vi "DAQ control panel.vi"() -> ()   [LabVIEW 2017]
uses:
  <vilib>/DAQmx/write.llb/DAQmx Write (Analog DBL 1Chan 1Samp).vi
  <vilib>/DAQmx/write.llb/DAQmx Write (Digital Bool 1Line 1Point).vi
  <vilib>/DAQmx/write.llb/DAQmx Write (Analog Wfm 1Chan NSamp).vi
  <vilib>/DAQmx/read.llb/DAQmx Read (Analog 1D DBL 1Chan NSamp).vi
  <vilib>/Analysis/baseanly.llb/Mean (DBL).vi
  <vilib>/DAQmx/read.llb/DAQmx Read (Analog 1D Wfm NChan NSamp).vi
  <vilib>/DAQmx/read.llb/DAQmx Read (Digital Bool 1Line 1Point).vi
  <vilib>/DAQmx/create/channels.llb/DAQmx Create Channel (AO-Voltage-Basic).vi
  <vilib>/DAQmx/miscellaneous.llb/DAQmx Fill In Error Info.vi
  <vilib>/DAQmx/create/channels.llb/DAQmx Create Channel (DO-Digital Output).vi
  <vilib>/DAQmx/create/channels.llb/DAQmx Create Channel (AI-Voltage-Basic).vi
  <vilib>/DAQmx/configure/timing.llb/DAQmx Timing (Sample Clock).vi
  <vilib>/measure/mascope.llb/Amplitude and Levels 1 chan.vi
  <vilib>/measure/mascope.llb/Pulse Measurements 1 chan.vi
  <vilib>/DAQmx/create/channels.llb/DAQmx Create Channel (DI-Digital Input).vi
  <vilib>/measure/NI_MABase.lvlib
  <vilib>/measure/NI_MAPro.lvlib
  <vilib>/Analysis/NI_AALBase.lvlib
panel:
  in  "Expected Input":bool
  out "ao1coerced?":bool caption="Output \nCoerced?"
  out "ao0coerced?":bool caption="Output \nCoerced?"
  in  "Set AO0":bool
  in  "AO0 phase":dbl
  in  "AO0 offset":dbl format="%0.2p"
  in  "AO0 sampling info":cluster{"Samples/sec":dbl, "# of Samples":dbl}={"Samples/sec"=1000000.0, "# of Samples"=1000000.0}
  in  "DC (Ch 0)":bool
  in  "AO0 signal type":T1(ring)
  in  "AO0 Frequency":dbl[unit]=1000.0
  in  "AO0 Amplitude":dbl[unit] min=-10.0 max=10.0
  out "DC offset":dbl[unit]
  out "frequency":dbl[unit]
  out "DC Voltage / Vpp":dbl[unit] format="%.2p"
  out "period":dbl[unit] format="%.2g"
  in  "# of samples":i32=1000
  in  "rate":dbl[unit]=1000.0 format="%0.2f"
  out "data":waveform(dbl)(graph)
  out "Digital Inputs":bool[](array[boolean])
  in  "Read Digital":bool
  in  "Digital toggle":bool[](array[boolean])=[FALSE, FALSE, FALSE, FALSE, FALSE, FALSE, FALSE, FALSE]
  in  "Digital Outputs":bool[](array[boolean])=[FALSE, FALSE, FALSE, FALSE, FALSE, FALSE, FALSE, FALSE]
  in  "physical channels":tag="Dev1/ai0"
  in  "Read Analog":bool
  in  "Set AO1":bool
  in  "AO1 phase":dbl
  in  "AO1 offset":dbl format="%0.2p"
  in  "AO1 sampling info":cluster{"Samples/sec":dbl, "# of Samples":dbl}={"Samples/sec"=1000000.0, "# of Samples"=1000000.0}
  in  "DC (Ch 1)":bool
  out "error out":errorcluster
  in  "error in (no error)":errorcluster
  in  "AO1 signal type":T1(ring)
  in  "AO1 Frequency":dbl[unit]=1000.0
  in  "AO1 Amplitude":dbl[unit] min=-10.0 max=10.0
  in  "stop":bool
  # "BNC-2120"
  # "7"
  # "7"
  # "7"
  # "6"
  # "6"
  # "6"
  # "5"
  # "5"
  # "5"
  # "AC"
  # "4"
  # "4"
  # "4"
  # "3"
  # "3"
  # "3"
  # "2"
  # "2"
  # "2"
  # "1"
  # "1"
  # "1"
  # "0"
  # "0"
  # "0"
  # "Output"
  # "Input"
  # "AC"
  # "DC"
  # "AC"
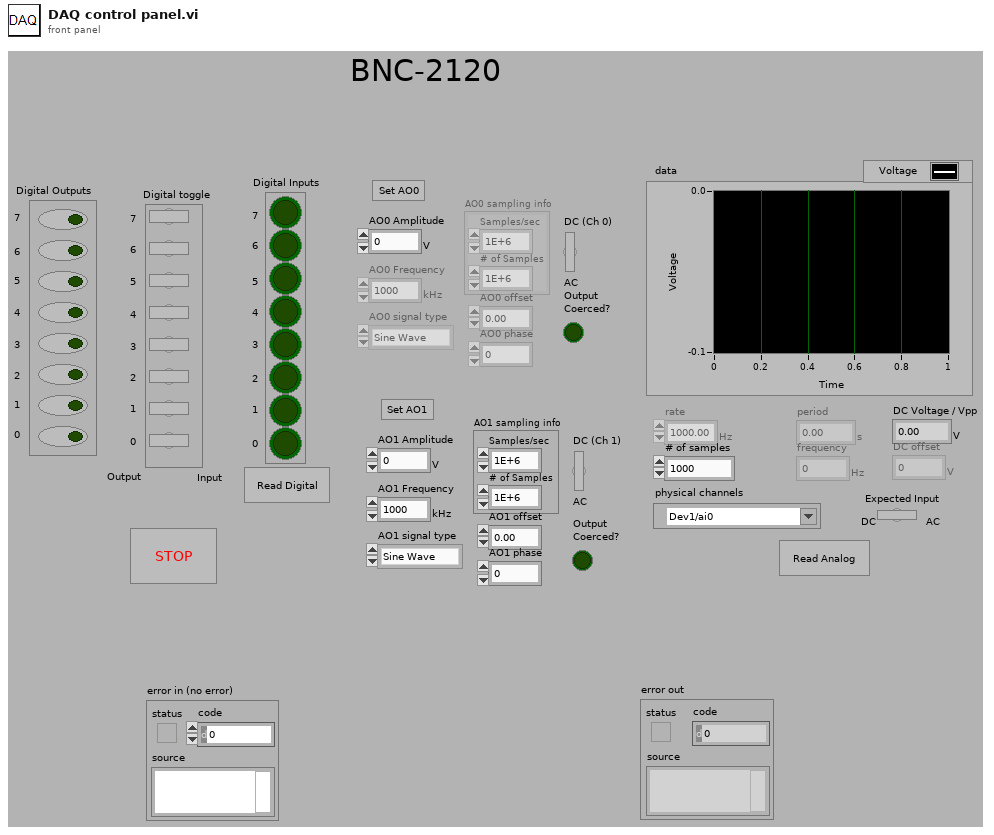
[diagram p1: front panel]
types:
  T1 = enum16{"Sine Wave", "Triangle Wave", "Square Wave", "Sawtooth Wave"}
  T2 = cluster{"AO ch0":refnum<k21>, "AO ch1":refnum<k21>}
  T3 = enum8{"Enabled", "Disabled", "Disabled and Grayed Out"}
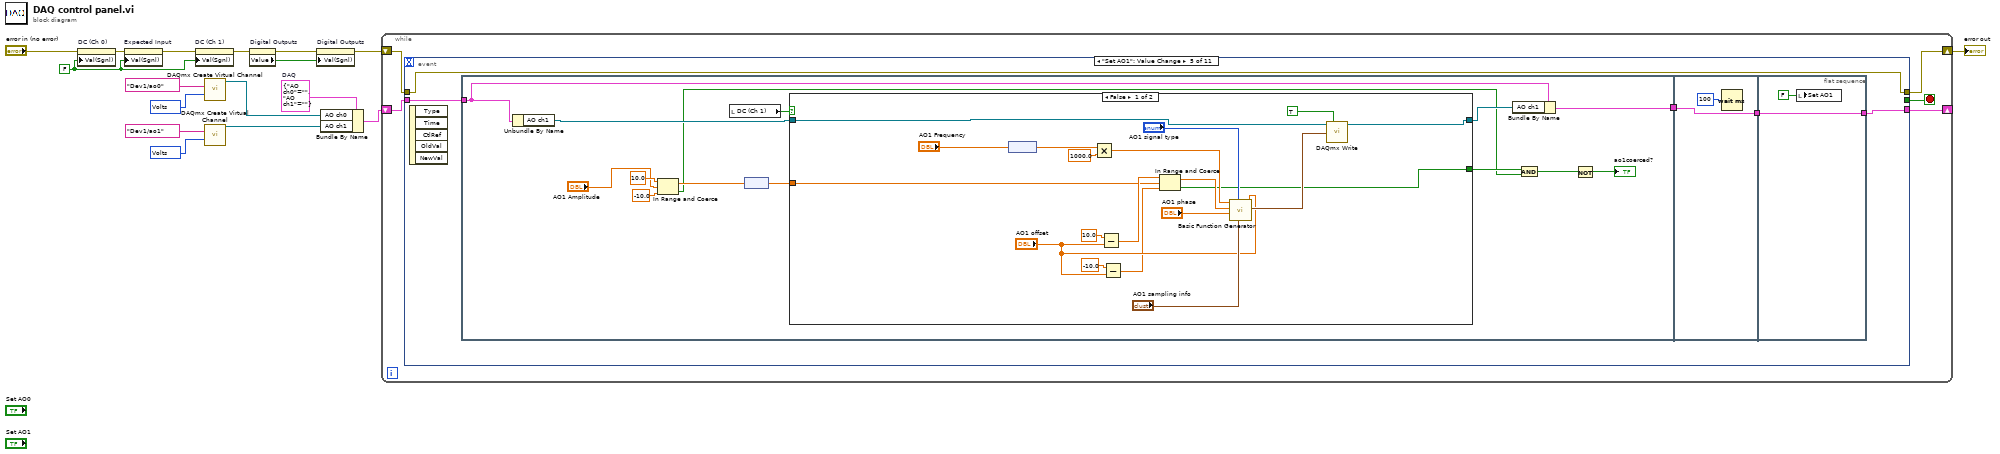
[diagram p0: block diagram]
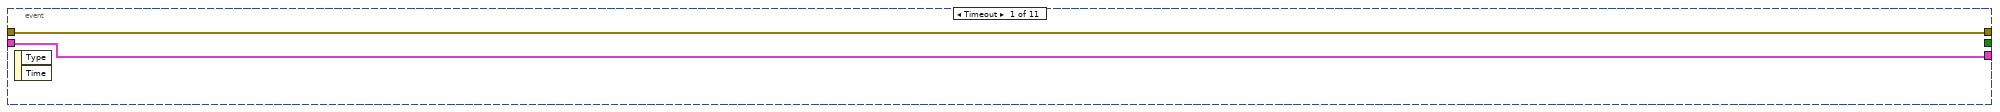
[diagram p2: hidden frame]
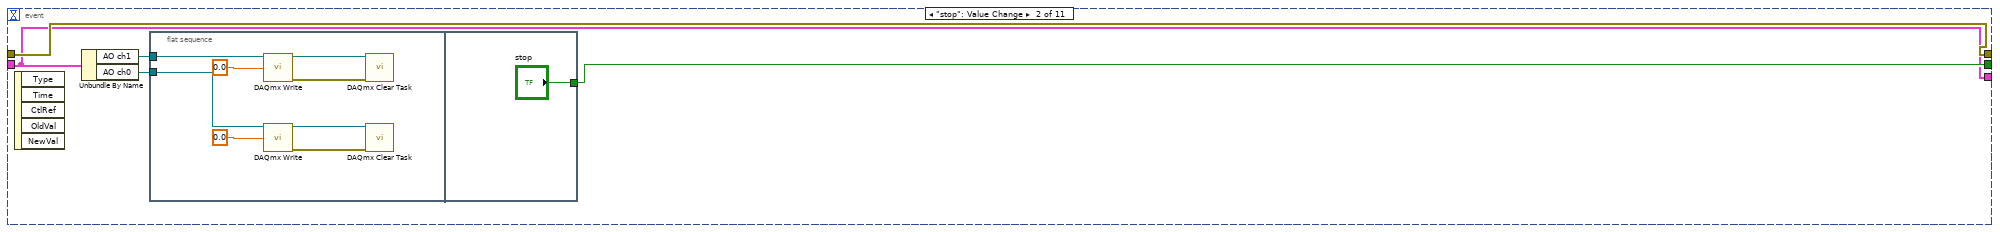
[diagram p3: hidden frame]
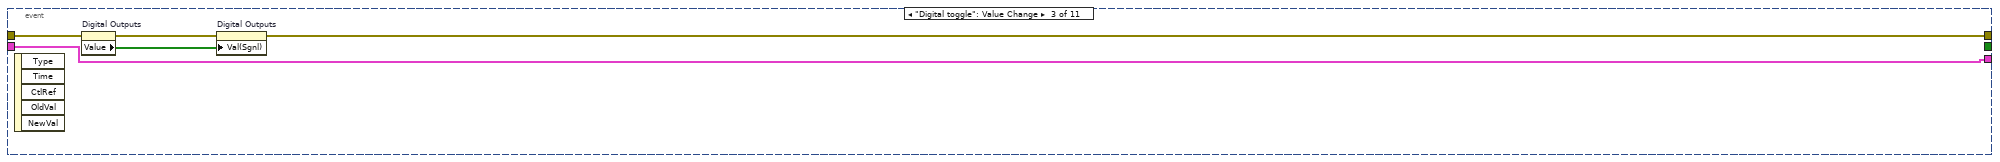
[diagram p4: hidden frame]
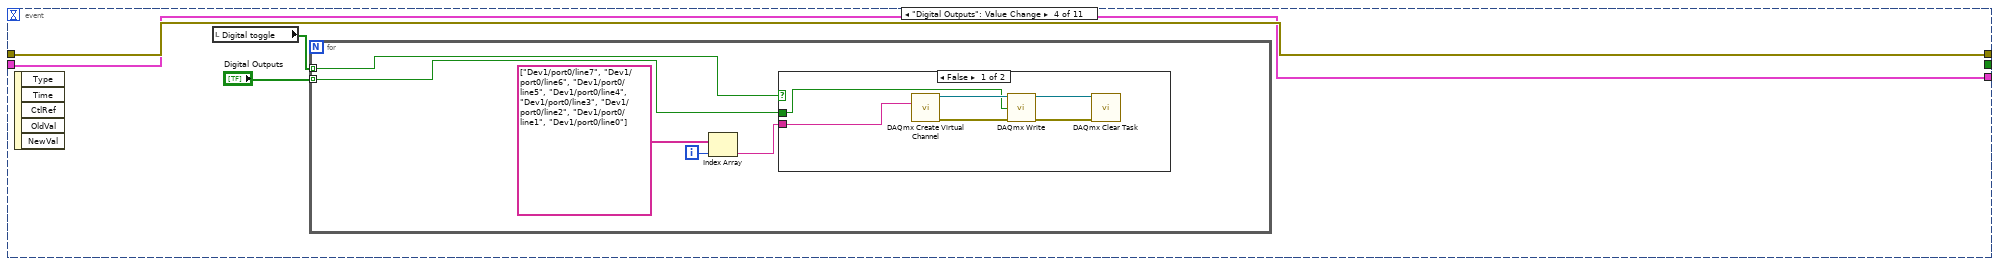
[diagram p5: hidden frame]
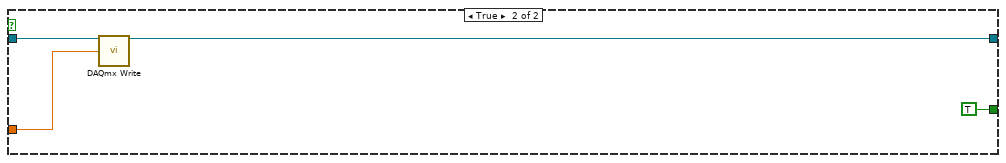
[diagram p7: hidden frame]
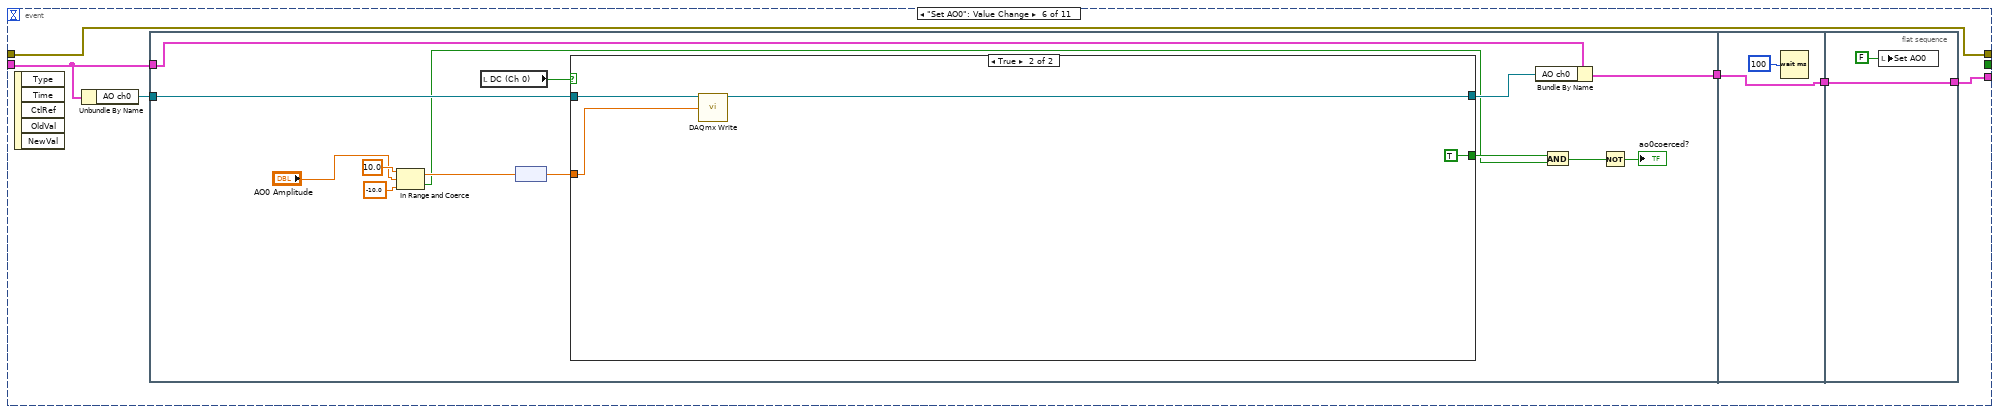
[diagram p8: hidden frame]
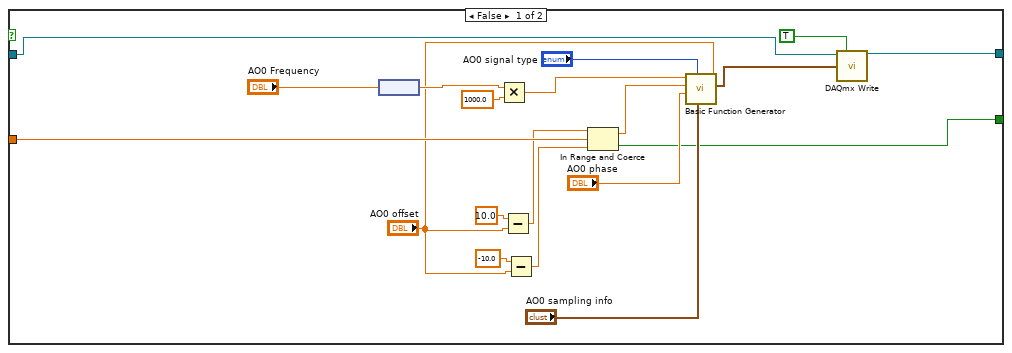
[diagram p9: hidden frame]
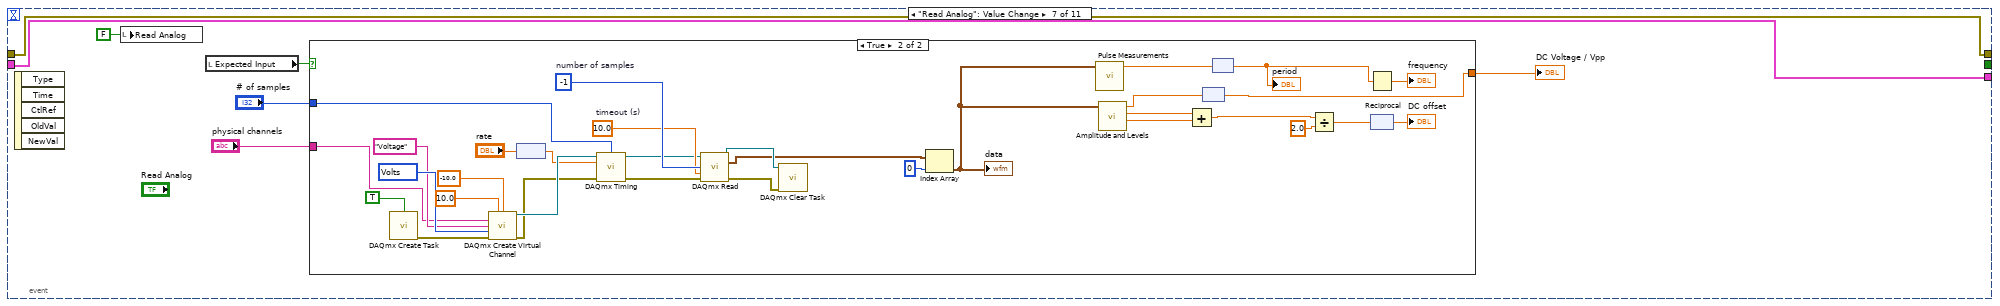
[diagram p10: hidden frame]
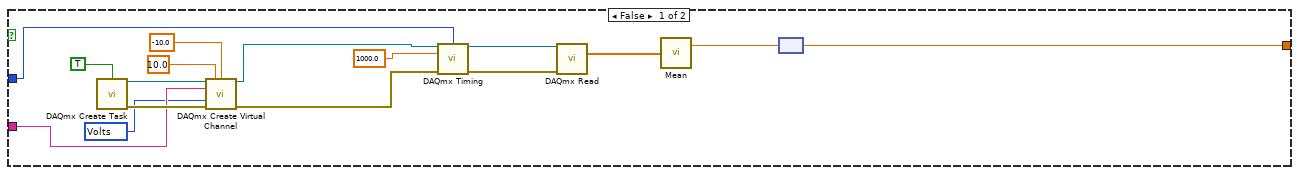
[diagram p11: hidden frame]
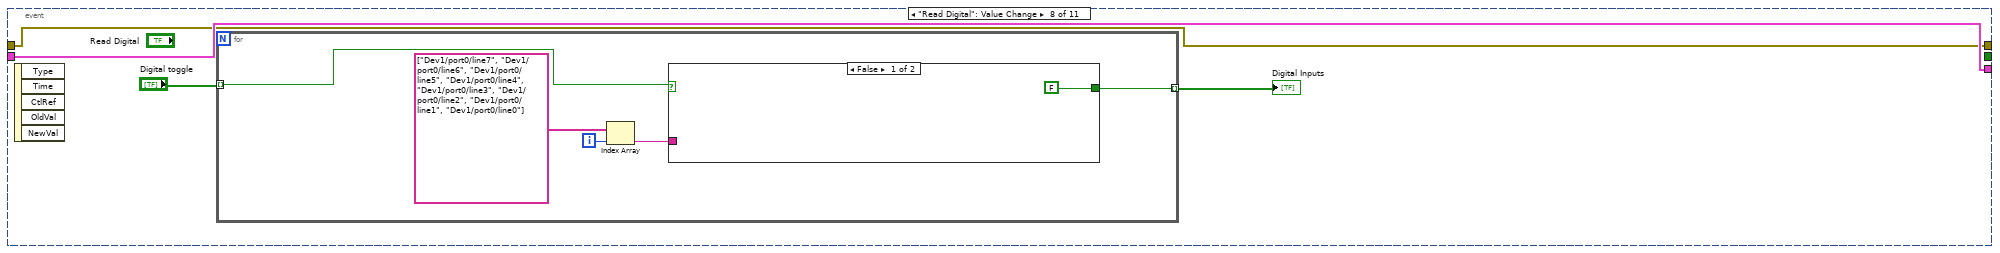
[diagram p12: hidden frame]
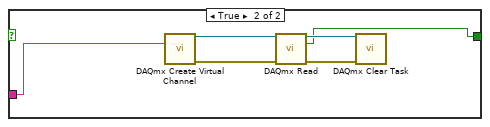
[diagram p13: hidden frame]
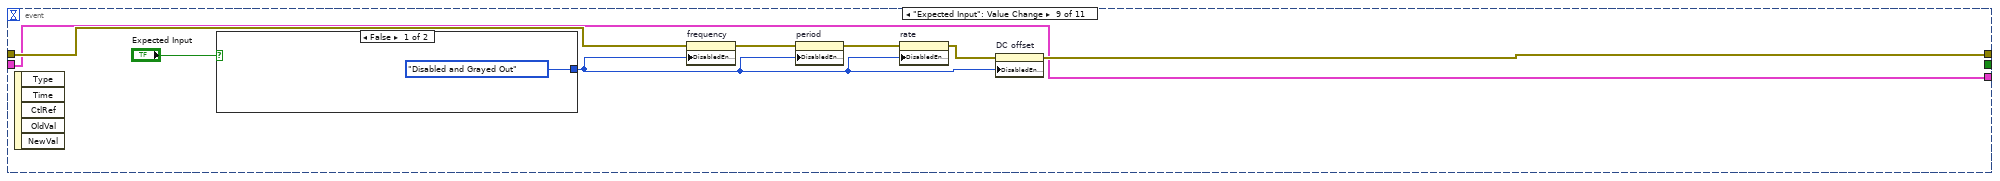
[diagram p14: hidden frame]
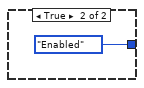
[diagram p15: hidden frame]
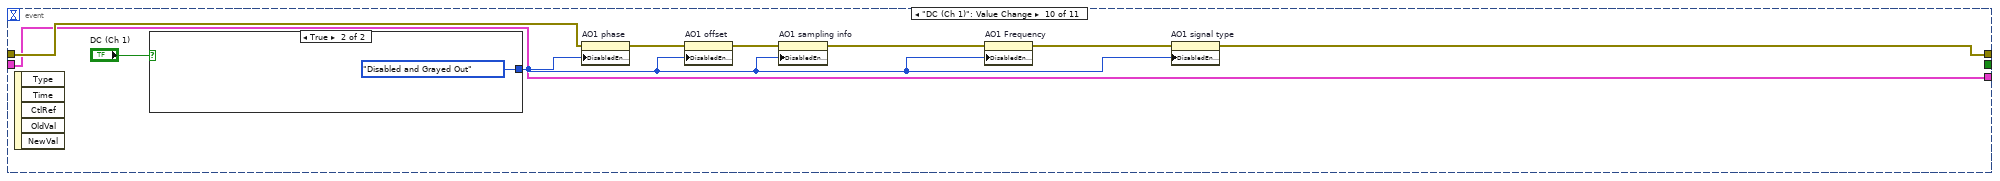
[diagram p16: hidden frame]
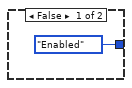
[diagram p17: hidden frame]
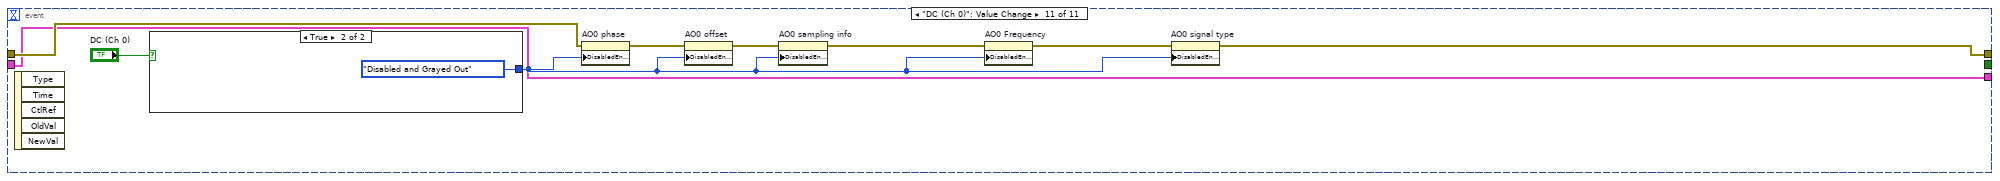
[diagram p18: hidden frame]
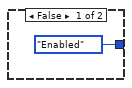
[diagram p19: hidden frame]
diagram:
  w12 = T2 {"AO ch0"="", "AO ch1"=""}  # DAQ
  w13 = 10348 items=["Volts"=10348, "From Custom Scale"=10065] ("units")
  w16 = 10348 items=["Volts"=10348, "From Custom Scale"=10065] ("units")
  w5 = FALSE ("DC (Ch 0)")
  n1 = property on="DC (Ch 0)" class="Bool (strict)"(error in="error in (no error)", "Val(Sgnl)"=w5) -> (error out=w6:errorcluster)  [unwired: 1 in, 1 out]
  n2 = property on="Expected Input" class="Bool (strict)"(error in=w6, "Val(Sgnl)"=w5) -> (error out=w7:errorcluster)  [unwired: 1 in, 1 out]
  n3 = property on="DC (Ch 1)" class="Bool (strict)"(error in=w7, "Val(Sgnl)"=w5) -> (error out=w2:errorcluster)  [unwired: 1 in, 1 out]
  n4 = call-poly <vilib>:"DAQmx Create Virtual Channel.vi"("physical channels"=tag "Dev1/ao0", "units"=w16) -> ("task out"=w10:refnum<k21>)  [unwired: 12 in, 1 out]
  n5 = call-poly <vilib>:"DAQmx Create Virtual Channel.vi"("physical channels"=tag "Dev1/ao1", "units"=w13) -> ("task out"=w11:refnum<k21>)  [unwired: 12 in, 1 out]
  n6 = property on="Digital Outputs" class="Arr (strict)"(error in=w2) -> (error out=w3:errorcluster, "Value"=w4:bool[])  [unwired: 1 in, 1 out]
  n7 = property on="Digital Outputs" class="Arr (strict)"(error in=w3, "Val(Sgnl)"=w4) -> (error out=w1:errorcluster)  [unwired: 1 in, 1 out]
  n8 = Bundle By Name(cluster=w12, "AO ch0"=w10, "AO ch1"=w11) -> (w9:T2)
  n9 = while {
    shift-right: [w20] -> w17
    shift-left: w1 -> [w21]
    shift-right: [w18] -> _
    shift-left: w9 -> [w19]
    stop <- w22 stop-if-true
    n10 = event shown="[4] \"Set AO1\": Value Change" {
      selector: _ -> [_ _ _ _ _ _ _ _ _ _ _]
      dyn-events: _ -> [_ _ _ _ _ _ _ _ _ _ _]
      timeout: _ -> [_ _ _ _ _ _ _ _ _ _ _]
      tunnel: [_ w29 _ _ _ _ _ _ _ _ _] -> w22
      tunnel: w21 -> [w24 w28 w40 w47 w63 w110 w157 w207 w230 w236 w247]
      tunnel: [w24 w28 w39 w47 w63 w110 w157 w207 w225 w237 w248] -> w20
      tunnel: w19 -> [w23 w27 w43 w44 w62 w108 w158 w208 w223 w234 w245]
      tunnel: [w23 w27 w43 w44 w61 w107 w158 w208 w223 w234 w245] -> w18
      event Timeout {
        n11 = event-data() -> ()  [unwired: 1 in, 2 out]
      }
      event "stop": Value Change {
        n12 = event-data() -> ()  [unwired: 1 in, 5 out]
        n13 = Unbundle By Name(w27) -> ("AO ch1"=w26:refnum<k21>, "AO ch0"=w25:refnum<k21>)
        n14 = flat-sequence {
          tunnel: w26 -> [w34]
          tunnel: w25 -> [w30]
          tunnel: ["stop"] -> w29
          frame #0 {
            n15 = call-poly <vilib>:"DAQmx Write.vi"("task/channels in"=w34, "data"=0.0) -> ("task out"=w37:refnum<k21>, "error out"=w36:errorcluster)  [unwired: 11 in, 1 out]
            n16 = call-poly <vilib>:"DAQmx Write.vi"("task/channels in"=w30, "data"=0.0) -> ("task out"=w31:refnum<k21>, "error out"=w32:errorcluster)  [unwired: 11 in, 1 out]
            n17 = call <vilib>:"DAQmx Clear Task.vi"("task in"=w37, "error in"=w36) -> ()  [unwired: 13 in, 1 out]
            n18 = call <vilib>:"DAQmx Clear Task.vi"("task in"=w31, "error in"=w32) -> ()  [unwired: 13 in, 1 out]
          }
          frame #1 {
          }
        }
      }
      event "Digital toggle": Value Change {
        n19 = event-data() -> ()  [unwired: 1 in, 5 out]
        n20 = property on="Digital Outputs" class="Arr (strict)"(error in=w40) -> (error out=w41:errorcluster, "Value"=w42:bool[])  [unwired: 1 in, 1 out]
        n21 = property on="Digital Outputs" class="Arr (strict)"(error in=w41, "Val(Sgnl)"=w42) -> (error out=w39:errorcluster)  [unwired: 1 in, 1 out]
      }
      event "Digital Outputs": Value Change {
        n22 = event-data() -> ()  [unwired: 1 in, 5 out]
        n23 = local read "Digital toggle"() -> (w45:bool[])
        n24 = for {
          tunnel: "Digital Outputs" -> [w48] mode=indexing
          tunnel: w45 -> [w49] mode=indexing
          i -> [w51]
          n25 = Index Array(array=tag[] ["Dev1/port0/line7", "Dev1/port0/line6", "Dev1/port0/line5", "Dev1/port0/line4", "Dev1/port0/line3", "Dev1/port0/line2", "Dev1/port0/line1", "Dev1/port0/line0"], index=w51) -> (element=w50:tag)
          n26 = case shown="False" w49 {
            tunnel: w50 -> [w58 _]
            tunnel: w48 -> [w55 _]
            frame False {
              n27 = call-poly <vilib>:"DAQmx Create Virtual Channel.vi"("lines"=w58) -> ("task out"=w57:refnum<k21>, "error out"=w56:errorcluster)  [unwired: 13 in]
              n28 = call-poly <vilib>:"DAQmx Write.vi"("task/channels in"=w57, "data"=w55, "error in"=w56) -> ("task out"=w54:refnum<k21>, "error out"=w53:errorcluster)  [unwired: 10 in, 1 out]
              n29 = call <vilib>:"DAQmx Clear Task.vi"("task in"=w54, "error in"=w53) -> ()  [unwired: 13 in, 1 out]
            }
            frame True {
            }
          }
        }
      }
      event "Set AO1": Value Change {
        n30 = event-data() -> ()  [unwired: 1 in, 5 out]
        n31 = flat-sequence {
          tunnel: w62 -> [w72]
          tunnel: [w71] -> w60
          tunnel: w60 -> [w102]
          tunnel: [w102] -> w59
          tunnel: [w104] -> w61
          tunnel: w59 -> [w104]
          frame #0 {
            n32 = Unbundle By Name(w72) -> ("AO ch1"=w76:refnum<k21>)
            n33 = In Range and Coerce(upper limit=dbl[unit] 10.0, x="AO1 Amplitude", lower limit=dbl[unit] -10.0) -> (coerced(x)=w73:dbl[unit], In Range?=w64:bool)
            n34 = local read "DC (Ch 1)"() -> (w68:bool)
            n35 = node(w73) -> (w77:dbl)
            n36 = case shown="False" w68 {
              tunnel: w76 -> [w78 w100]
              tunnel: w77 -> [w83 w99]
              tunnel: [w89 w98] -> w70
              tunnel: [w79 TRUE] -> w65
              frame False {
                n37 = node("AO1 Frequency") -> (w95:dbl)
                n38 = Multiply(x=w95, y=1000.0) -> (x*y=w87:dbl)
                n39 = Subtract(x=10.0, y="AO1 offset") -> (x-y=w86:dbl)
                n40 = Subtract(x=-10.0, y="AO1 offset") -> (x-y=w81:dbl)
                n41 = In Range and Coerce(upper limit=w86, x=w83, lower limit=w81) -> (coerced(x)=w80:dbl, In Range?=w79:bool)
                n42 = call <vilib>:"Basic Function Generator.vi"("offset"="AO1 offset", "sampling info"="AO1 sampling info", "signal type"="AO1 signal type", "phase"="AO1 phase", "amplitude"=w80, "frequency"=w87) -> ("signal out"=w94:waveform(dbl))  [unwired: 3 in, 2 out]
                n43 = call-poly <vilib>:"DAQmx Write.vi"("task/channels in"=w78, "auto start"=TRUE, "data"=w94) -> ("task out"=w89:refnum<k21>)  [unwired: 10 in, 2 out]
              }
              frame True {
                n44 = call-poly <vilib>:"DAQmx Write.vi"("task/channels in"=w100, "data"=w99) -> ("task out"=w98:refnum<k21>)  [unwired: 11 in, 2 out]
              }
            }
            n45 = Bundle By Name(cluster=w72, "AO ch1"=w70) -> (w71:T2)
            n46 = And(x=w65, y=w64) -> (x .and. y?=w66:bool)
            n47 = Not(x=w66) -> (.not. x?=→"ao1coerced?":bool)
          }
          frame #1 {
            n48 = Wait (ms)(milliseconds to wait=u32 100) -> ()  [unwired: 1 out]
          }
          frame #2 {
            n49 = local write "Set AO1"(FALSE ("Set AO1")) -> ()
          }
        }
      }
      event "Set AO0": Value Change {
        n50 = event-data() -> ()  [unwired: 1 in, 5 out]
        n51 = Unbundle By Name(w108) -> ("AO ch0"=w109:refnum<k21>)
        n52 = flat-sequence {
          tunnel: w109 -> [w123]
          tunnel: w108 -> [w119]
          tunnel: [w118] -> w106
          tunnel: w106 -> [w149]
          tunnel: [w149] -> w105
          tunnel: [w151] -> w107
          tunnel: w105 -> [w151]
          frame #0 {
            n53 = In Range and Coerce(upper limit=dbl[unit] 10.0, x="AO0 Amplitude", lower limit=dbl[unit] -10.0) -> (coerced(x)=w120:dbl[unit], In Range?=w113:bool)
            n54 = local read "DC (Ch 0)"() -> (w115:bool)
            n55 = node(w120) -> (w124:dbl)
            n56 = case shown="True" w115 {
              tunnel: w123 -> [w139 w147]
              tunnel: w124 -> [w132 w146]
              tunnel: [w138 w145] -> w117
              tunnel: [w125 TRUE] -> w114
              frame False {
                n57 = node("AO0 Frequency") -> (w142:dbl)
                n58 = Multiply(x=w142, y=1000.0) -> (x*y=w133:dbl)
                n59 = Subtract(x=10.0, y="AO0 offset") -> (x-y=w131:dbl)
                n60 = Subtract(x=-10.0, y="AO0 offset") -> (x-y=w129:dbl)
                n61 = In Range and Coerce(upper limit=w131, x=w132, lower limit=w129) -> (coerced(x)=w126:dbl, In Range?=w125:bool)
                n62 = call <vilib>:"Basic Function Generator.vi"("offset"="AO0 offset", "sampling info"="AO0 sampling info", "signal type"="AO0 signal type", "phase"="AO0 phase", "amplitude"=w126, "frequency"=w133) -> ("signal out"=w141:waveform(dbl))  [unwired: 3 in, 2 out]
                n63 = call-poly <vilib>:"DAQmx Write.vi"("task/channels in"=w139, "auto start"=TRUE, "data"=w141) -> ("task out"=w138:refnum<k21>)  [unwired: 10 in, 2 out]
              }
              frame True {
                n64 = call-poly <vilib>:"DAQmx Write.vi"("task/channels in"=w147, "data"=w146) -> ("task out"=w145:refnum<k21>)  [unwired: 11 in, 2 out]
              }
            }
            n65 = Bundle By Name(cluster=w119, "AO ch0"=w117) -> (w118:T2)
            n66 = And(x=w114, y=w113) -> (x .and. y?=w112:bool)
            n67 = Not(x=w112) -> (.not. x?=→"ao0coerced?":bool)
          }
          frame #1 {
            n68 = Wait (ms)(milliseconds to wait=u32 100) -> ()  [unwired: 1 out]
          }
          frame #2 {
            n69 = local write "Set AO0"(FALSE ("Set AO1")) -> ()
          }
        }
      }
      event "Read Analog": Value Change {
        n70 = event-data() -> ()  [unwired: 1 in, 5 out]
        n71 = local write "Read Analog"(FALSE ("Read AI")) -> ()
        n72 = local read "Expected Input"() -> (w153:bool)
        n73 = case shown="True" w153 {
          tunnel: "physical channels" -> [w167 w177]
          tunnel: [w160 w176] -> w154
          tunnel: "# of samples" -> [w159 w175]
          frame False {
            w162 = 10348 items=["Volts"=10348, "From Custom Scale"=10065] ("units")
            n74 = call <vilib>:"DAQmx Create Task.vi"("auto cleanup"=TRUE) -> ("task out"=w173:refnum<k21>, "error out"=w170:errorcluster)  [unwired: 13 in]
            n75 = call-poly <vilib>:"DAQmx Create Virtual Channel.vi"("task in"=w173, "maximum value"=10.0, "minimum value"=-10.0, "physical channels"=w167, "units"=w162, "error in"=w170) -> ("task out"=w169:refnum<k21>, "error out"=w168:errorcluster)  [unwired: 8 in]
            n76 = call-poly <vilib>:"DAQmx Timing.vi"("task/channels in"=w169, "samples per channel"=w159, "rate"=1000.0, "error in"=w168) -> ("task out"=w165:refnum<k21>, "error out"=w164:errorcluster)  [unwired: 10 in]
            n77 = call-poly <vilib>:"DAQmx Read.vi"("task/channels in"=w165, "error in"=w164) -> ("data"=w163:dbl[])  [unwired: 11 in, 2 out]
            n78 = call-poly <vilib>:"Mean.vi"("X"=w163) -> ("mean"=w161:dbl)  [unwired: 1 out]
            n79 = node(w161) -> (w160:dbl[unit])
          }
          frame True {
            w200 = 10348 items=["Volts"=10348, "From Custom Scale"=10065] ("units")
            w205 = 10.0  # timeout (s)
            w206 = -1  # number of samples
            n80 = call <vilib>:"DAQmx Create Task.vi"("auto cleanup"=TRUE) -> ("error out"=w201:errorcluster)  [unwired: 13 in, 1 out]
            n81 = call-poly <vilib>:"DAQmx Create Virtual Channel.vi"("maximum value"=10.0, "minimum value"=-10.0, "physical channels"=w177, "name to assign"="Voltage", "units"=w200, "error in"=w201) -> ("task out"=w196:refnum<k21>, "error out"=w195:errorcluster)  [unwired: 8 in]
            n82 = node("rate") -> (w186:dbl)
            n83 = call-poly <vilib>:"DAQmx Timing.vi"("task/channels in"=w196, "samples per channel"=w175, "rate"=w186, "error in"=w195) -> ("task out"=w194:refnum<k21>, "error out"=w193:errorcluster)  [unwired: 10 in]
            n84 = call-poly <vilib>:"DAQmx Read.vi"("task/channels in"=w194, "number of samples per channel"=w206, "timeout"=w205, "error in"=w193) -> ("task out"=w203:refnum<k21>, "data"=w192:waveform(dbl)[], "error out"=w204:errorcluster)  [unwired: 9 in]
            n85 = call <vilib>:"DAQmx Clear Task.vi"("task in"=w203, "error in"=w204) -> ()  [unwired: 13 in, 1 out]
            n86 = Index Array(array=w192, index=0) -> (element=w190:waveform(dbl))
            "data" <- w190
            n87 = call-poly <vilib>:"Pulse Measurements.vi"("signal in"=w190) -> ("period"=w189:dbl)  [unwired: 6 in, 4 out]
            n88 = call-poly <vilib>:"Amplitude and Levels.vi"("signal in"=w190) -> ("low state level"=w182:dbl, "high state level"=w183:dbl, "amplitude"=w188:dbl)  [unwired: 7 in, 1 out]
            n89 = Add(x=w183, y=w182) -> (x+y=w181:dbl)
            n90 = node(w188) -> (w176:dbl[unit])
            n91 = node(w189) -> (w185:dbl[unit])
            "period" <- w185
            n92 = Divide(x=w181, y=2.0) -> (x/y=w179:dbl)
            n93 = Reciprocal(x=w185) -> (1/x=→"frequency":dbl[unit])
            n94 = node(w179) -> (→"DC offset":dbl[unit])
          }
        }
        "DC Voltage / Vpp" <- w154
      }
      event "Read Digital": Value Change {
        n95 = event-data() -> ()  [unwired: 1 in, 5 out]
        n96 = for {
          tunnel: "Digital toggle" -> [w211] mode=indexing
          tunnel: [w212] -> w209 mode=indexing
          i -> [w214]
          n97 = Index Array(array=tag[] ["Dev1/port0/line7", "Dev1/port0/line6", "Dev1/port0/line5", "Dev1/port0/line4", "Dev1/port0/line3", "Dev1/port0/line2", "Dev1/port0/line1", "Dev1/port0/line0"], index=w214) -> (element=w213:tag)
          n98 = case shown="False" w211 {
            tunnel: w213 -> [_ w221]
            tunnel: [FALSE w217] -> w212
            frame False {
            }
            frame True {
              n99 = call-poly <vilib>:"DAQmx Create Virtual Channel.vi"("lines"=w221) -> ("task out"=w222:refnum<k21>, "error out"=w220:errorcluster)  [unwired: 13 in]
              n100 = call-poly <vilib>:"DAQmx Read.vi"("task/channels in"=w222, "error in"=w220) -> ("task out"=w218:refnum<k21>, "data"=w217:bool, "error out"=w219:errorcluster)  [unwired: 11 in]
              n101 = call <vilib>:"DAQmx Clear Task.vi"("task in"=w218, "error in"=w219) -> ()  [unwired: 13 in, 1 out]
            }
          }
        }
        "Digital Inputs" <- w209
      }
      event "Expected Input": Value Change {
        n102 = event-data() -> ()  [unwired: 1 in, 5 out]
        n103 = case shown="False" "Expected Input" {
          tunnel: [T3."Disabled and Grayed Out" ("Disabled") T3."Enabled" ("Disabled")] -> w226
          frame False {
          }
          frame True {
          }
        }
        n104 = property on="frequency" class="DigNum (strict)"(error in=w230, "DisabledEnum"=w226) -> (error out=w229:errorcluster)  [unwired: 1 in, 1 out]
        n105 = property on="period" class="DigNum (strict)"(error in=w229, "DisabledEnum"=w226) -> (error out=w228:errorcluster)  [unwired: 1 in, 1 out]
        n106 = property on="rate" class="DigNum (strict)"(error in=w228, "DisabledEnum"=w226) -> (error out=w227:errorcluster)  [unwired: 1 in, 1 out]
        n107 = property on="DC offset" class="DigNum (strict)"(error in=w227, "DisabledEnum"=w226) -> (error out=w225:errorcluster)  [unwired: 1 in, 1 out]
      }
      event "DC (Ch 1)": Value Change {
        n108 = event-data() -> ()  [unwired: 1 in, 5 out]
        n109 = case shown="True" "DC (Ch 1)" {
          tunnel: [T3."Enabled" ("Disabled") T3."Disabled and Grayed Out" ("Disabled")] -> w235
          frame False {
          }
          frame True {
          }
        }
        n110 = property on="AO1 phase" class="DigNum (strict)"(error in=w236, "DisabledEnum"=w235) -> (error out=w238:errorcluster)  [unwired: 1 in, 1 out]
        n111 = property on="AO1 offset" class="DigNum (strict)"(error in=w238, "DisabledEnum"=w235) -> (error out=w239:errorcluster)  [unwired: 1 in, 1 out]
        n112 = property on="AO1 sampling info" class="Clust (strict)"(error in=w239, "DisabledEnum"=w235) -> (error out=w240:errorcluster)  [unwired: 1 in, 1 out]
        n113 = property on="AO1 Frequency" class="DigNum (strict)"(error in=w240, "DisabledEnum"=w235) -> (error out=w241:errorcluster)  [unwired: 1 in, 1 out]
        n114 = property on="AO1 signal type" class="Enum (strict)"(error in=w241, "DisabledEnum"=w235) -> (error out=w237:errorcluster)  [unwired: 1 in, 1 out]
      }
      event "DC (Ch 0)": Value Change {
        n115 = event-data() -> ()  [unwired: 1 in, 5 out]
        n116 = case shown="True" "DC (Ch 0)" {
          tunnel: [T3."Enabled" ("Disabled") T3."Disabled and Grayed Out" ("Disabled")] -> w246
          frame False {
          }
          frame True {
          }
        }
        n117 = property on="AO0 phase" class="DigNum (strict)"(error in=w247, "DisabledEnum"=w246) -> (error out=w249:errorcluster)  [unwired: 1 in, 1 out]
        n118 = property on="AO0 offset" class="DigNum (strict)"(error in=w249, "DisabledEnum"=w246) -> (error out=w250:errorcluster)  [unwired: 1 in, 1 out]
        n119 = property on="AO0 sampling info" class="Clust (strict)"(error in=w250, "DisabledEnum"=w246) -> (error out=w251:errorcluster)  [unwired: 1 in, 1 out]
        n120 = property on="AO0 Frequency" class="DigNum (strict)"(error in=w251, "DisabledEnum"=w246) -> (error out=w252:errorcluster)  [unwired: 1 in, 1 out]
        n121 = property on="AO0 signal type" class="Enum (strict)"(error in=w252, "DisabledEnum"=w246) -> (error out=w248:errorcluster)  [unwired: 1 in, 1 out]
      }
    }
  }
  "error out" <- w17
